vi "readKey.vi"(6 "Error in":errorcluster, 7 "Table Name":string, 8 "Value":dbl format="%#_13g", 9 "Found?":bool, 10 "Refnum in":T1, 11 "Key Name":string) -> (0 "error out":errorcluster, 2 "Warning":string, 3 "value":dbl)   [LabVIEW 2014]
uses:
  <vilib>/Utility/config.llb/Config Data RefNum.ctl
  <vilib>/Utility/config.llb/Write Key (Double).vi
  <vilib>/Utility/config.llb/NI_LVConfig.lvlib
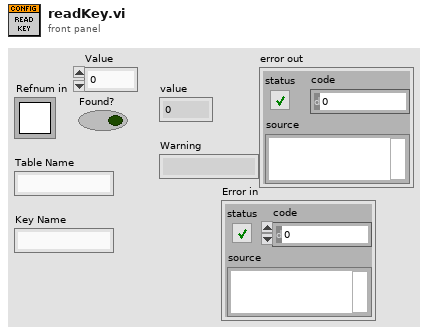
[diagram p1: front panel]
types:
  T1 = typedef "NI_LVConfig.lvlib/Config Data RefNum.ctl" = refnum<k1>
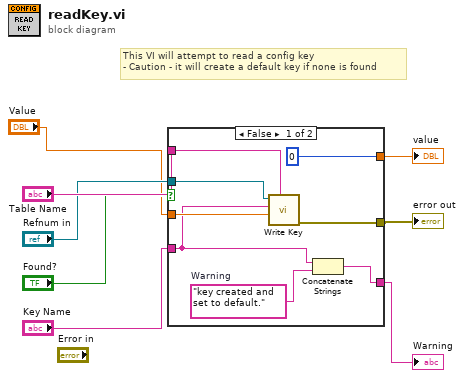
[diagram p0: block diagram]
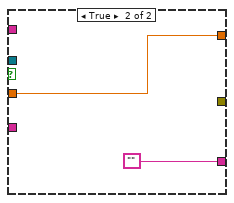
[diagram p2: hidden frame]
diagram:
  # "This VI will attempt to read a config key \n- Caution - it will create a default key if none is found"
  n1 = case shown="False" "Found?" {
    tunnel: "Refnum in" -> [w16 _]
    tunnel: "Key Name" -> [w10 _]
    tunnel: "Value" -> [w13 w18]
    tunnel: "Table Name" -> [w15 _]
    tunnel: [w14 _] -> w2
    tunnel: [0 ("value") w18] -> w7
    tunnel: [w9 ""] -> w8
    frame False {
      w11 = "key created and set to default."  # Warning
      n2 = call-poly <vilib>:"Write Key.vi"("section"=w15, "value"=w13, "key"=w10, "refnum"=w16) -> ("error out"=w14:errorcluster)  [unwired: 5 in, 2 out]
      n3 = Concatenate Strings(w10, w11) -> (w9:string)
    }
    frame True {
    }
  }
  "Warning" <- w8
  "value" <- w7
  "error out" <- w2
